vi "PLC Puck.vi"(11 "PVT":T1={"Mode"=1, "Pressure PV"=0.0, "Pressure SP"=0.0, "Flow PV"=0.0, "Flow SP"=0.0, "Volume PV"=0.0, "Volume SP"=0.0, "MM PV"=0.0, "Start"=FALSE, "Home"=FALSE} {"MM PV" scale format="%#.2f"; "Volume SP" format="%.3f"; "Volume PV" format="%.3f"; "Flow SP" format="%.3f"; "Flow PV" format="%.3f"; "Pressure SP" format="%.3f"; "Pressure PV" format="%.3f"; "Mode" items=["Давление"=1, "Расход"=2, "Объём"=3, "Извлечение"=4]}) -> (3 "appended array":u16[](array[numeric]))   [LabVIEW 2023, in "Drive.lvlib"]
uses:
  Drive.lvlib
  PVT_Drive_Type.ctl
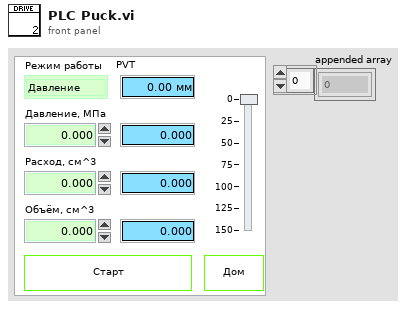
[diagram p1: front panel]
types:
  T1 = typedef "Drive.lvlib/PVT_Drive_Type.ctl" = cluster{"Mode":u16, "Pressure PV":dbl, "Pressure SP":dbl, "Flow PV":dbl, "Flow SP":dbl, "Volume PV":dbl, "Volume SP":dbl, "MM PV":dbl, "Start":bool, "Home":bool}
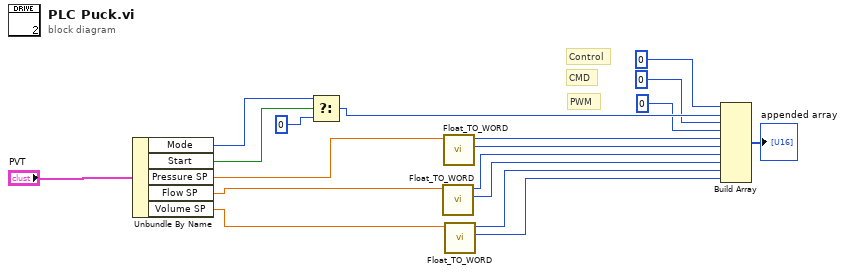
[diagram p0: block diagram]
diagram:
  # "CMD"
  # "PWM"
  # "Control"
  n1 = Unbundle By Name("PVT") -> ("Mode"=w16:u16, "Start"=w17:bool, "Pressure SP"=w10:dbl, "Flow SP"=w9:dbl, "Volume SP"=w8:dbl)
  n2 = Select(t=w16, s=w17, f=u16 0) -> (s? t:f=w13:u16)
  n3 = call "Float_TO_WORD.vi"("FLOAT"=w9) -> ("second_Word"=w4:u16, "first_Word"=w5:u16)  [unwired: 9 in]
  n4 = call "Float_TO_WORD.vi"("FLOAT"=w10) -> ("second_Word"=w6:u16, "first_Word"=w7:u16)  [unwired: 9 in]
  n5 = call "Float_TO_WORD.vi"("FLOAT"=w8) -> ("second_Word"=w2:u16, "first_Word"=w3:u16)  [unwired: 9 in]
  n6 = Build Array(u16 0 ("f"), w13, u16 0 ("f"), u16 0 ("f"), w7, w6, w5, w4, w3, w2) -> (→"appended array":u16[])
